vi "Simple Digital Output.vi"() -> ()   [LabVIEW 2025]
doc: "Simple Digital Output\n\nThis example shows how to write an output to a digital channel.\n\nThis example expects a USB cable connected from your development PC to the Type B USB Jack (next to the power input) on the roboRIO."
uses:
  <vilib>/Rock Robotics/SystemInterfaces/DIO/FPGA_DIOChannel.ctl
panel:
  in  "DIOChannel":T1=enum."DIO 7"
  in  "stop":bool
  in  "Digital Value":bool
  # "Set this input before running."
  # "This can be set while running."
  # "_"
  # "(   )"
  # "Output Signal"
  # "(+)"
  # "This shows the wiring for an output signal.  When the Digital Value switch is turned on, the Output Signal should read +5VDC between (+) and (-)."
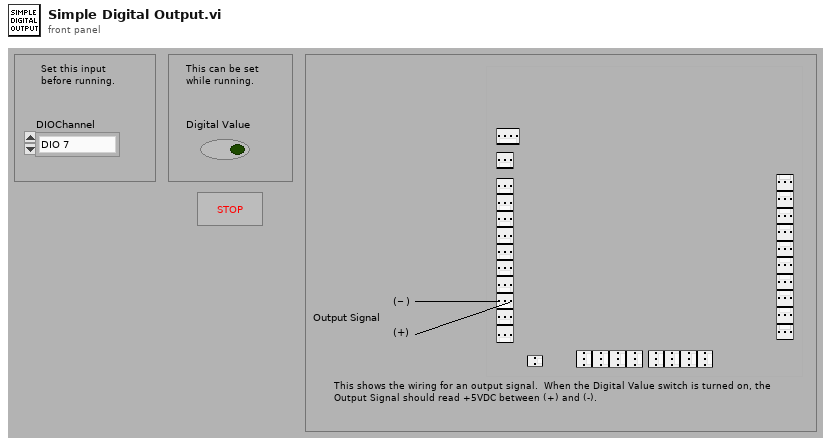
[diagram p1: front panel]
types:
  T1 = typedef "FPGA_DIOChannel.ctl" = enum8{"DIO 0", "DIO 1", "DIO 2", "DIO 3", "DIO 4", "DIO 5", "DIO 6", "DIO 7", "DIO 8", "DIO 9", "DIO MXP 0", "DIO MXP 1", "DIO MXP 2", "DIO MXP 3", "DIO MXP 4", "DIO MXP 5", "DIO MXP 6", "DIO MXP 7", "DIO MXP 8", "DIO MXP 9", "DIO MXP 10", "DIO MXP 11", "DIO MXP 12", "DIO MXP 13", "DIO MXP 14", "DIO MXP 15", "SPI Port CS1", "SPI Port CS2", "SPI Port CS3", "SPI Port MISO", "SPI Port MOSI", "Invalid"}
  T2 = typedef "WPI_DigitalOutputDevRef.ctl" = cluster{"DIO Channel":T1, "DevStatus":errorcluster}
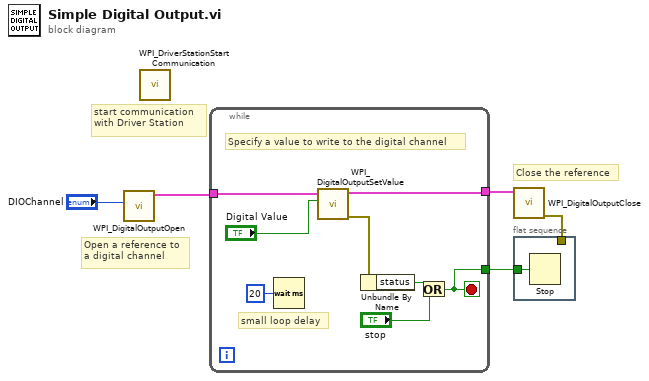
[diagram p0: block diagram]
diagram:
  # "start communication with Driver Station"
  # "Close the reference"
  # "Open a reference to\na digital channel"
  n1 = call <vilib>:"WPI_DigitalOutputOpen.vi"("DIO Channel"="DIOChannel") -> ("DigitalOutputDevRef"=w4:T2)  [unwired: 1 in, 9 out]
  n2 = call <vilib>:"WPI_DriverStationStart Communication.vi"() -> ()  [unwired: 3 in, 9 out]
  n3 = while {
    tunnel: w4 -> [w13]
    tunnel: [w11] -> w3
    tunnel: [w8] -> w1
    stop <- w8 stop-if-true
    # "small loop delay"
    # "Specify a value to write to the digital channel"
    n4 = Wait (ms)(milliseconds to wait=u32 20) -> ()  [unwired: 1 out]
    n5 = call <vilib>:"WPI_DigitalOutputSetValue.vi"("Value"="Digital Value", "DigitalOutputDevRef"=w13) -> ("error out"=w10:errorcluster, "DigitalOutputDevRef"=w11:T2)  [unwired: 1 in, 7 out]
    n6 = Unbundle By Name(w10) -> ("status"=w9:bool)
    n7 = Or(x=w9, y="stop") -> (x .or. y?=w8:bool)
  }
  n8 = call <vilib>:"WPI_DigitalOutputClose.vi"("DigitalOutputDevRef"=w3) -> ("error out"=w2:errorcluster)  [unwired: 1 in, 9 out]
  n9 = flat-sequence {
    tunnel: w2 -> [_]
    tunnel: w1 -> [w14]
    frame #0 {
      n10 = Stop(stop? (T)=w14) -> ()
    }
  }
